vi "Read Place point.vi"(8 "error in (no error)":errorcluster, 11 "Control in":refnum<class "Control.lvclass">) -> (0 "error out":errorcluster, 1 "Text Point":cluster{"x":i32, "y":i32}, 2 "Point":cluster{"x":i32, "y":i32}, 3 "Control out":refnum<class "Control.lvclass">)   [LabVIEW 2013, in "uitools_Control.lvlib" / "Control.lvclass"]
uses:
  Control.lvclass
  Control.lvclass/Control.ctl
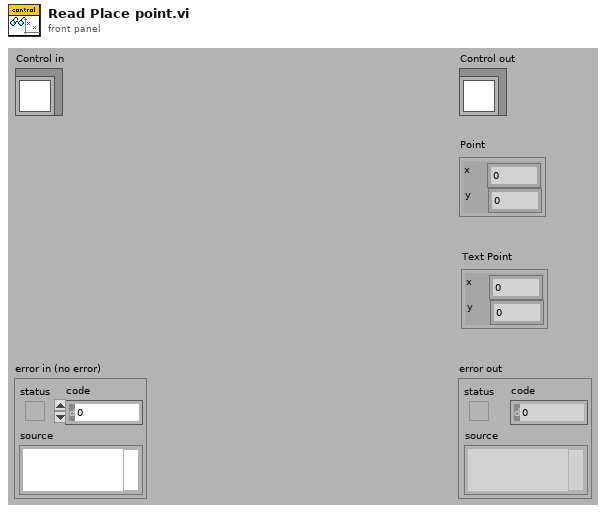
[diagram p1: front panel]
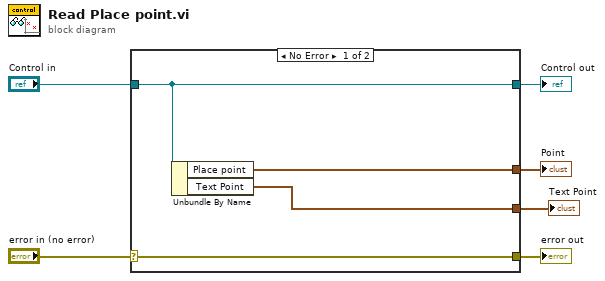
[diagram p0: block diagram]
diagram:
  n1 = case shown="No Error" "error in (no error)" {
    selector: "error in (no error)" -> [w10 w11]
    tunnel: [w10 w11] -> w5
    tunnel: [w9 w12] -> w3
    tunnel: "Control in" -> [w9 w12]
    tunnel: [w8 _] -> w2
    tunnel: [w7 _] -> w1
    frame No Error {
      n2 = Unbundle By Name(w9) -> ("Place point"=w8:cluster{"x":i32, "y":i32}, "Text Point"=w7:cluster{"x":i32, "y":i32})
    }
    frame Error {
    }
  }
  "error out" <- w5
  "Control out" <- w3
  "Point" <- w2
  "Text Point" <- w1
